vi "Tosca-Initialize Digital Outputs.vi"(0 "Imaging":T1, 7 "Fs (Hz)":dbl, 9 "Npts":i32, 11 "error in (no error)":errorcluster) -> (4 "Digital Outputs":string[](array[string]), 6 "DO":T3, 15 "error out":errorcluster)   [LabVIEW 2020]
uses:
  Typedefs/Tosca-DO Runtime.ctl
  Typedefs/Tosca-Imaging.ctl
  Imaging VIs/Tosca-Imaging Mode.ctl
  epl-vi-lib/Connection VIs/Type Defs/CM-IO Type.ctl
  Tosca-Globals.vi
  epl-vi-lib/Utility VIs/Array Manipulation VIs/Sort and Index (string).vi
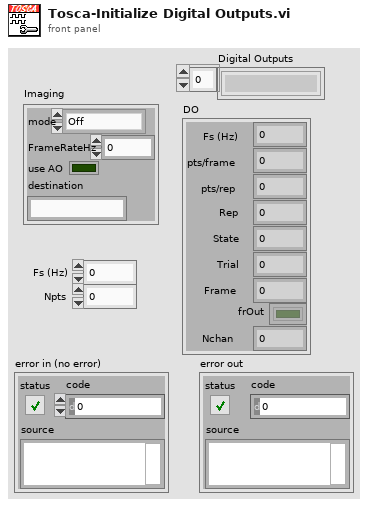
[diagram p1: front panel]
types:
  T1 = typedef "Tosca-Imaging.ctl" = cluster{"mode":T2, "FrameRateHz":dbl, "use AO":bool, "destination":string}
  T2 = typedef "Tosca-Imaging Mode.ctl" = enum16{"Off", "Widefield", "Two-photon"}
  T3 = typedef "Tosca-DO Runtime.ctl" = cluster{"Fs (Hz)":dbl, "pts/frame":i32, "pts/rep":i32, "Rep":i32, "State":i32, "Trial":i32, "Frame":i32, "frOut":bool[], "Nchan":i32}
  T4 = typedef "CM-IO Type.ctl" = enum16{"Analog Outputs", "Analog Inputs", "Digital Outputs", "Digital Inputs"}
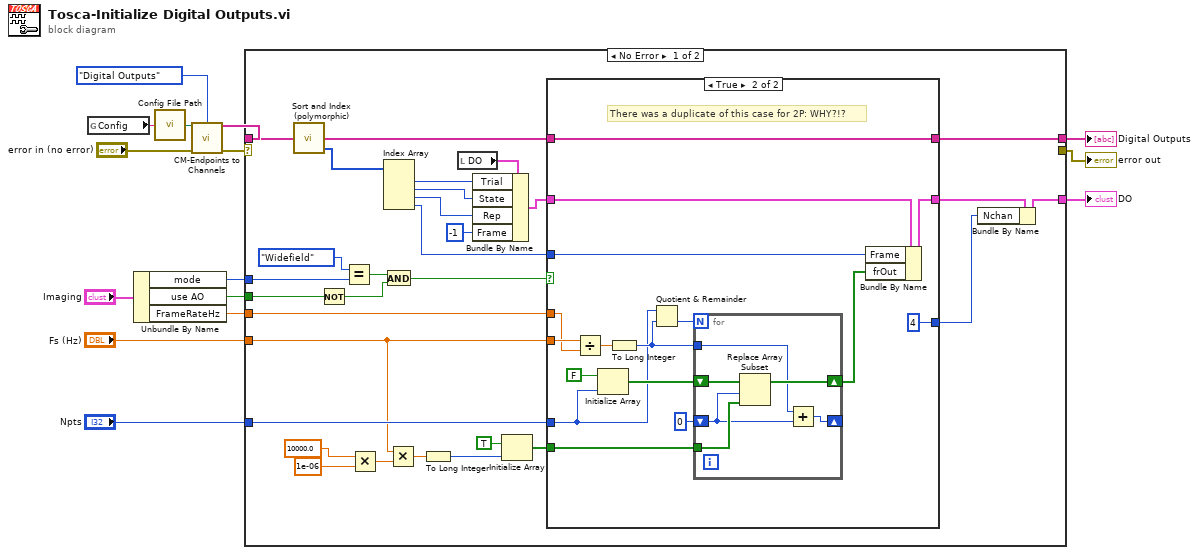
[diagram p0: block diagram]
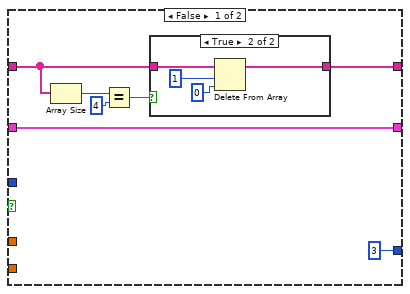
[diagram p2: hidden frame]
diagram:
  n1 = global read "Tosca-Globals.vi" "Config"() -> (w2:string)
  n2 = Unbundle By Name("Imaging") -> ("mode"=w1:T2, "use AO"=w12:bool, "FrameRateHz"=w11:dbl)
  n3 = call "Config File Path.vi"("AppName"=w2) -> ("Default config file name"=w7:path)
  n4 = call "CM-Endpoints to Channels.vi"("Path"=w7, "IO Type"=CM-IO_Type."Digital Outputs" ("Section"), "error in (no error)"="error in (no error)") -> ("IO Channels"=w4:string[], "error out"=w5:errorcluster)  [unwired: 11 in]
  n5 = case shown="No Error" w5 {
    selector: w5 -> [_ w80]
    tunnel: w4 -> [w45 _]
    tunnel: [w22 _] -> w15
    tunnel: [w39 _] -> w14
    tunnel: [_ w80] -> w13
    tunnel: w12 -> [w18 _]
    tunnel: w11 -> [w41 _]
    tunnel: "Fs (Hz)" -> [w31 _]
    tunnel: "Npts" -> [w37 _]
    tunnel: w1 -> [w21 _]
    frame No Error {
      n6 = call-poly "Sort and Index (polymorphic).vi"("X"=w45) -> ("Index"=w24:i32[], "Sort(X)"=w23:string[])  [unwired: 3 in]
      n7 = Not(x=w18) -> (.not. x?=w16:bool)
      n8 = Equal?(x=Tosca-Imaging_Mode."Widefield", y=w21) -> (x = y?=w19:bool)
      n9 = Multiply(x=10000.0, y=1e-06) -> (x*y=w33:dbl)
      n10 = Index Array(array=w24) -> (element #1=w27:i32, element #2=w26:i32, element #3=w25:i32, element #4=w28:i32)  [unwired: 4 in]
      n11 = And(x=w19, y=w16) -> (x .and. y?=w17:bool)
      n12 = Multiply(x=w31, y=w33) -> (x*y=w34:dbl)
      n13 = To Long Integer(number=w34) -> (32bit integer=w35:i32)
      n14 = local read "DO"() -> (w44:T3)
      n15 = Bundle By Name(cluster=w44, "Trial"=w27, "State"=w26, "Rep"=w25, "Frame"=-1) -> (w43:T3)
      n16 = Initialize Array(TRUE, w35) -> (w30:bool[])
      n17 = case shown="True" w17 {
        tunnel: w43 -> [w52 w73]
        tunnel: [w52 w72] -> w42
        tunnel: w28 -> [_ w71]
        tunnel: w41 -> [_ w69]
        tunnel: w31 -> [_ w70]
        tunnel: [3 4] -> w38
        tunnel: w37 -> [_ w60]
        tunnel: w30 -> [_ w63]
        tunnel: w23 -> [w47 w58]
        tunnel: [w46 w58] -> w22
        frame False {
          n18 = Array Size(array=w47) -> (size(s)=w50:i32)
          n19 = Equal?(x=w50, y=4) -> (x = y?=w48:bool)
          n20 = case shown="True" w48 {
            tunnel: w47 -> [w53 w57]
            tunnel: [w53 w56] -> w46
            frame False {
            }
            frame True {
              n21 = Delete From Array(array=w57, length=1, index=0) -> (array with subset deleted=w56:string[])  [unwired: 1 out]
            }
          }
        }
        frame True {
          # "There was a duplicate of this case for 2P: WHY?!?"
          n22 = Divide(x=w70, y=w69) -> (x/y=w68:dbl)
          n23 = Initialize Array(FALSE, w60) -> (w65:bool[])
          n24 = To Long Integer(number=w68) -> (32bit integer=w61:i32)
          n25 = Quotient & Remainder(x=w60, y=w61) -> (floor(x/y)=w59:i32)  [unwired: 1 out]
          n26 = for {
            N: w59 -> [_]
            shift-right: [w78] -> w64
            shift-left: w65 -> [w79]
            tunnel: w63 -> [w77]
            shift-right: [w75] -> _
            shift-left: 0 -> [w76]
            tunnel: w61 -> [w74]
            n27 = Replace Array Subset(array=w79, new element=w77, index=w76) -> (w78:bool[])
            n28 = Add(x=w74, y=w76) -> (x+y=w75:i32)
          }
          n29 = Bundle By Name(cluster=w73, "Frame"=w71, "frOut"=w64) -> (w72:T3)
        }
      }
      n30 = Bundle By Name(cluster=w42, "Nchan"=w38) -> (w39:T3)
    }
    frame Error {
    }
  }
  "DO" <- w14
  "Digital Outputs" <- w15
  "error out" <- w13
